vi "Read DAQ Type.vi"(8 "error in (no error)":errorcluster, 11 "PXIe 6363 in":refnum<class "PXIe 6363.lvclass">) -> (0 "error out":errorcluster, 2 "DAQ Type":enum16{"Hardware", "Simulation"}(ring), 3 "PXIe 6363 out":refnum<class "PXIe 6363.lvclass">)   [LabVIEW 2021, in "DAQ Hardware.lvlib" / "PXIe 6363.lvclass"]
uses:
  PXIe 6363.lvclass
  PXIe 6363.lvclass/PXIe 6363.ctl
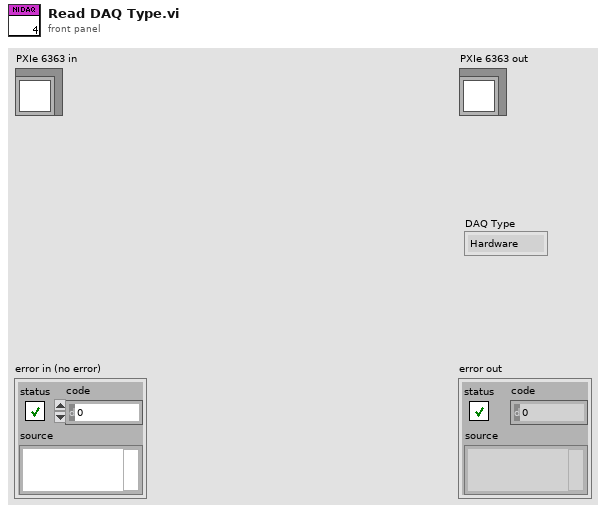
[diagram p1: front panel]
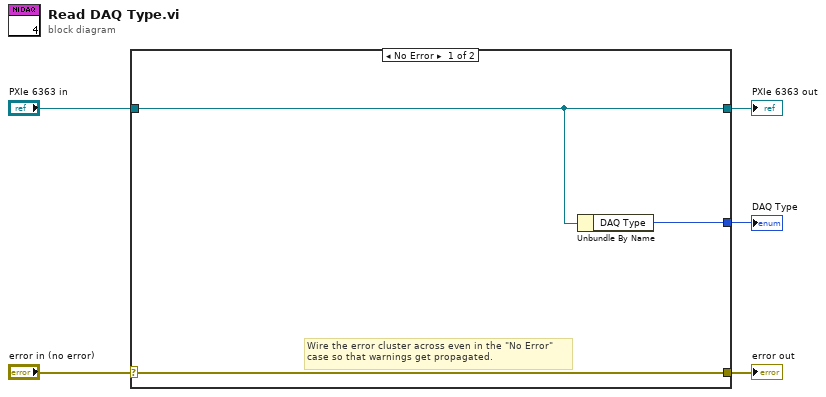
[diagram p0: block diagram]
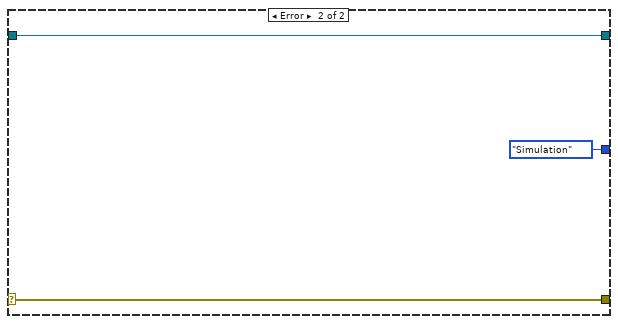
[diagram p2: hidden frame]
diagram:
  n1 = case shown="No Error" "error in (no error)" {
    selector: "error in (no error)" -> [w8 w11]
    tunnel: [w8 w11] -> w4
    tunnel: [w7 w10] -> w2
    tunnel: "PXIe 6363 in" -> [w7 w10]
    tunnel: [w6 enum16{"Hardware", "Simulation"}."Simulation" ("DAQ Type")] -> w1
    frame No Error {
      # "Wire the error cluster across even in the \"No Error\"\ncase so that warnings get propagated."
      n2 = Unbundle By Name(w7) -> ("DAQ Type"=w6:enum16{"Hardware", "Simulation"})
    }
    frame Error {
    }
  }
  "error out" <- w4
  "PXIe 6363 out" <- w2
  "DAQ Type" <- w1
